vi "Open Class.vi"(6 "Variant in":variant, 7 "Shift Pressed?":bool, 8 "error in (no error)":errorcluster, 10 "QD Combo Box Ref":refnum<vi>, 11 "QD Launch VI Ref":refnum<vi>) -> (0 "error out":errorcluster, 4 "Variant out":variant)   [LabVIEW 2020]
doc: "Finds a class in the selection (wire, terminal, control, subVI, etc), and opens it. If nothing is selected it opens the current VI's library.\n\nDefault Shortcut - [O]"
uses:
  <vilib>/Utility/traverseref.llb/VI Scripting - Traverse.lvlib
  <vilib>/Utility/traverseref.llb/TRef TravTarget.ctl
panel:
  # "Do not change the connector pane of this VI.\n\nSee the block diagram for directions on how to use this template."
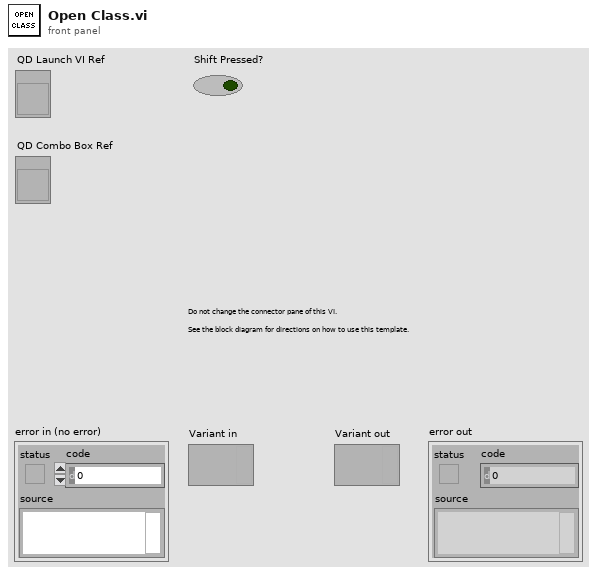
[diagram p1: front panel]
types:
  T1 = typedef "TRef TravTarget.ctl" = enum16{"FP", "BD", "Other"}
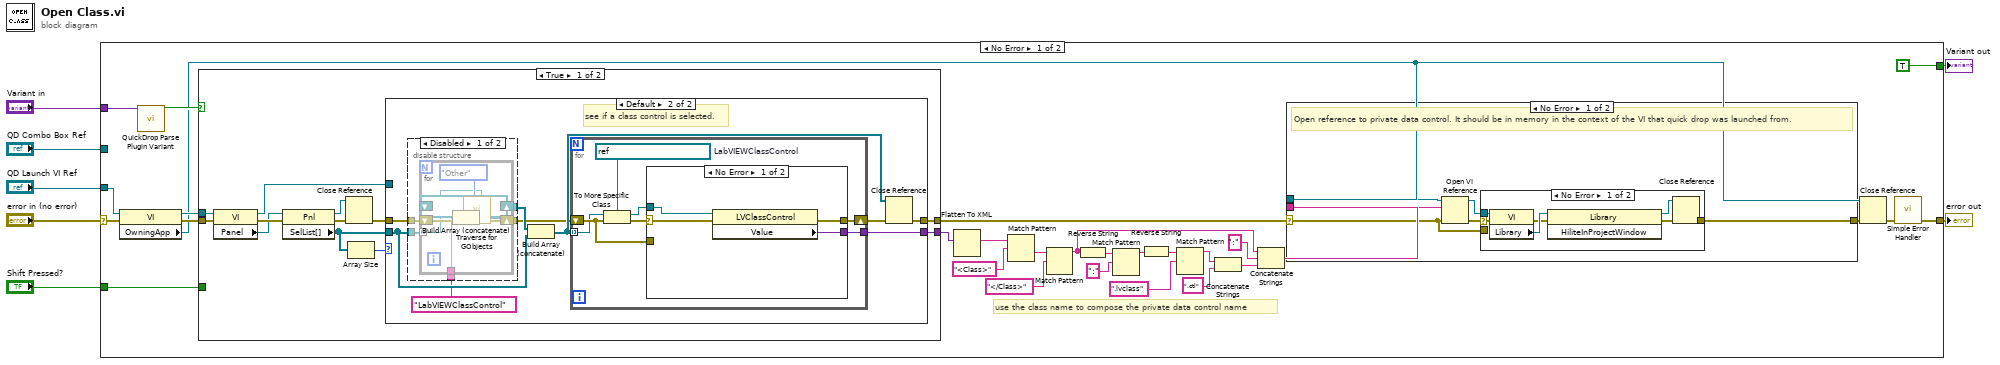
[diagram p0: block diagram]
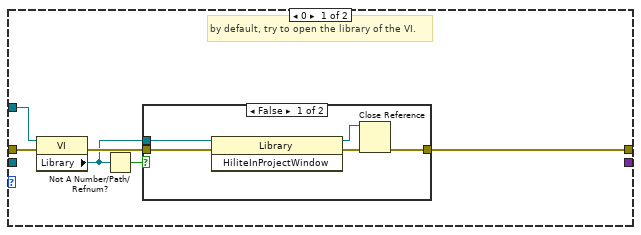
[diagram p4: hidden frame]
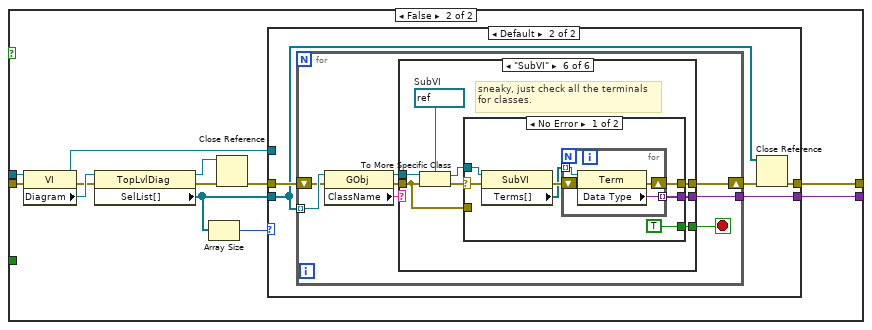
[diagram p8: hidden frame]
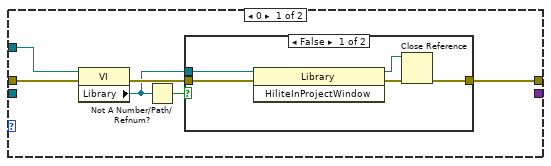
[diagram p9: hidden frame]
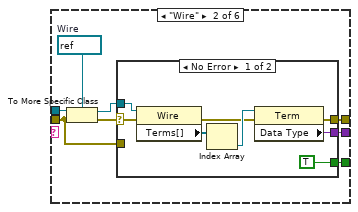
[diagram p12: hidden frame]
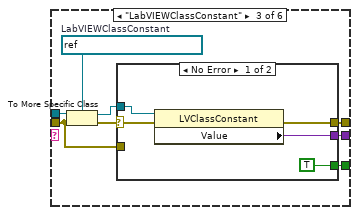
[diagram p14: hidden frame]
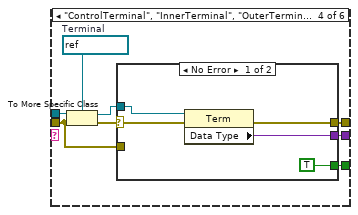
[diagram p16: hidden frame]
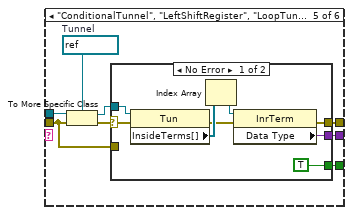
[diagram p18: hidden frame]
diagram:
  n1 = case shown="No Error" "error in (no error)" {
    selector: "error in (no error)" -> [w30 w232]
    tunnel: [w27 w232] -> w6
    tunnel: "QD Launch VI Ref" -> [w32 _]
    tunnel: "Shift Pressed?" -> [w34 _]
    tunnel: "QD Combo Box Ref" -> [_ _]
    tunnel: "Variant in" -> [w36 _]
    tunnel: [TRUE _] -> w1
    frame No Error {
      # "use the class name to compose the private data control name"
      n2 = property class="VI"(reference=w32, error in=w30) -> (reference out=w31:refnum<vi>, error out=w29:errorcluster, "OwningApp"=w8:refnum<vi>)
      n3 = call <vilib>:"QuickDrop Parse Plugin Variant.vi"("QDKS Variant in"=w36) -> ("QD Launch VI Panel?"=w33:bool)  [unwired: 12 in, 2 out]
      n4 = case shown="True" w33 {
        tunnel: w29 -> [w63 w123]
        tunnel: [w62 w122] -> w10
        tunnel: w34 -> [_ _]
        tunnel: w31 -> [w61 w121]
        tunnel: [w58 w116] -> w11
        frame True {
          n5 = property class="VI"(reference=w61, error in=w63) -> (reference out=w55:refnum<vi>, error out=w60:errorcluster, "Panel"=w59:refnum<vi>)
          n6 = property class="Pnl"(reference=w59, error in=w60) -> (reference out=w54:refnum<vi>, error out=w53:errorcluster, "SelList[]"=w56:refnum<vi>[])
          n7 = Close Reference(reference=w54, error in (no error)=w53) -> (error out=w52:errorcluster)
          n8 = Array Size(array=w56) -> (size(s)=w57:i32)
          n9 = case shown="Default" w57 {
            tunnel: [w65 w84] -> w62
            tunnel: w52 -> [w68 w82]
            tunnel: w56 -> [_ w80]
            tunnel: [_ w77] -> w58
            tunnel: w55 -> [w69 _]
            frame 0 {
              # "by default, try to open the library of the VI."
              n10 = property class="VI"(reference=w69, error in=w68) -> (error out=w66:errorcluster, "Library"=w64:refnum<vi>)  [unwired: 1 out]
              n11 = Not A Number/Path/Refnum?(number/path/refnum=w64) -> (NaN/Path/Refnum?=w67:bool)
              n12 = case shown="False" w67 {
                tunnel: w66 -> [w74 w75]
                tunnel: [w71 w75] -> w65
                tunnel: w64 -> [w70 _]
                frame False {
                  n13 = invoke class="Library" method="HiliteInProjectWindow"(reference=w70, error in=w74) -> (reference out=w72:refnum<vi>, error out=w73:errorcluster)  [unwired: 1 in, 1 out]
                  n14 = Close Reference(reference=w72, error in (no error)=w73) -> (error out=w71:errorcluster)
                }
                frame True {
                }
              }
            }
            frame Default {
              # "see if a class control is selected."
              n15 = disable-structure shown="Disabled" {
                disable-tunnel: [w90 w99] -> w76
                disable-tunnel: w82 -> [w89 w99]
                disable-tunnel: [w88 _] -> w81
                disable-tunnel: w80 -> [w87 _]
                disable-tunnel: "LabVIEWClassControl" ("Class Name") -> [w86 _]
                frame Disabled {
                  n16 = for {
                    shift-right: [w96] -> w90
                    shift-left: w89 -> [w95]
                    tunnel: w87 -> [w94] mode=indexing
                    tunnel: w86 -> [w93]
                    shift-right: [w91] -> w88
                    shift-left: refnum<vi>[] [] ("References") -> [w92]
                    n17 = call <vilib>:"Traverse for GObjects.vi"("Other Refnum"=w94, "Traverse Target"=TRef_TravTarget."Other", "error in (no error)"=w95, "Class Name"=w93) -> ("error out"=w96:errorcluster, "References"=w97:refnum<vi>[])  [unwired: 4 in, 2 out]
                    n18 = Build Array (concatenate)(w92, w97) -> (w91:refnum<vi>[])
                  }
                }
                frame Enabled {
                }
              }
              n19 = Build Array (concatenate)(w81, w80) -> (w83:refnum<vi>[])
              n20 = for {
                shift-right: [w106] -> w78
                shift-left: w76 -> [w103]
                tunnel: w83 -> [w102] mode=indexing
                tunnel: [w100] -> w77
                w101 = refnum<vi> refnum  # LabVIEWClassControl
                n21 = To More Specific Class(target class=w101, reference=w102, error in=w103) -> (specific class reference=w105:refnum<vi>, error out=w104:errorcluster)
                n22 = case shown="No Error" w104 {
                  selector: w104 -> [w110 _]
                  tunnel: [w109 w111] -> w106
                  tunnel: w105 -> [w108 _]
                  tunnel: w103 -> [_ w111]
                  tunnel: [w107 _] -> w100
                  frame No Error {
                    n23 = property class="LVClassControl"(reference=w108, error in=w110) -> (error out=w109:errorcluster, "Value"=w107:variant)  [unwired: 1 out]
                  }
                  frame Error {
                  }
                }
              }
              n24 = Close Reference(reference=w83, error in (no error)=w78) -> (error out=w84:errorcluster)
            }
          }
        }
        frame False {
          n25 = property class="VI"(reference=w121, error in=w123) -> (reference out=w112:refnum<vi>, error out=w119:errorcluster, "Diagram"=w120:refnum<vi>)
          n26 = property class="TopLvlDiag"(reference=w120, error in=w119) -> (reference out=w118:refnum<vi>, error out=w115:errorcluster, "SelList[]"=w114:refnum<vi>[])
          n27 = Array Size(array=w114) -> (size(s)=w113:i32)
          n28 = Close Reference(reference=w118, error in (no error)=w115) -> (error out=w117:errorcluster)
          n29 = case shown="Default" w113 {
            tunnel: [w126 w140] -> w122
            tunnel: w117 -> [w127 w139]
            tunnel: [_ w137] -> w116
            tunnel: w114 -> [_ w136]
            tunnel: w112 -> [w125 _]
            frame 0 {
              n30 = property class="VI"(reference=w125, error in=w127) -> (error out=w129:errorcluster, "Library"=w128:refnum<vi>)  [unwired: 1 out]
              n31 = Not A Number/Path/Refnum?(number/path/refnum=w128) -> (NaN/Path/Refnum?=w124:bool)
              n32 = case shown="False" w124 {
                tunnel: w129 -> [w134 w135]
                tunnel: [w131 w135] -> w126
                tunnel: w128 -> [w130 _]
                frame False {
                  n33 = invoke class="Library" method="HiliteInProjectWindow"(reference=w130, error in=w134) -> (reference out=w132:refnum<vi>, error out=w133:errorcluster)  [unwired: 1 in, 1 out]
                  n34 = Close Reference(reference=w132, error in (no error)=w133) -> (error out=w131:errorcluster)
                }
                frame True {
                }
              }
            }
            frame Default {
              n35 = for {
                shift-right: [w148] -> w138
                shift-left: w139 -> [w144]
                tunnel: w136 -> [w145] mode=indexing
                tunnel: [w146] -> w137
                stop <- w147 stop-if-true
                n36 = property class="GObj"(reference=w145, error in=w144) -> (reference out=w142:refnum<vi>, error out=w143:errorcluster, "ClassName"=w141:string)
                n37 = case shown="\"SubVI\"" w141 {
                  tunnel: [w149 w155 w173 w187 w201 w218] -> w148
                  tunnel: [_ w153 w171 w185 w199 w216] -> w147
                  tunnel: [_ w152 w170 w184 w198 w215] -> w146
                  tunnel: w143 -> [w149 w151 w169 w183 w197 w214]
                  tunnel: w142 -> [_ w150 w168 w182 w196 w213]
                  frame Default {
                  }
                  frame "Wire" {
                    w157 = refnum<vi> refnum  # Wire
                    n38 = To More Specific Class(target class=w157, reference=w150, error in=w151) -> (specific class reference=w154:refnum<vi>, error out=w156:errorcluster)
                    n39 = case shown="No Error" w156 {
                      selector: w156 -> [w165 _]
                      tunnel: [w160 w166] -> w155
                      tunnel: w154 -> [w164 _]
                      tunnel: w151 -> [_ w166]
                      tunnel: [TRUE _] -> w153
                      tunnel: [w158 _] -> w152
                      frame No Error {
                        n40 = property class="Wire"(reference=w164, error in=w165) -> (error out=w161:errorcluster, "Terms[]"=w163:refnum<vi>[])  [unwired: 1 out]
                        n41 = Index Array(array=w163) -> (element=w162:refnum<vi>)  [unwired: 1 in]
                        n42 = property class="Term"(reference=w162, error in=w161) -> (error out=w160:errorcluster, "Data Type"=w158:variant)  [unwired: 1 out]
                      }
                      frame Error {
                      }
                    }
                  }
                  frame "LabVIEWClassConstant" {
                    w167 = refnum<vi> refnum  # LabVIEWClassConstant
                    n43 = To More Specific Class(target class=w167, reference=w168, error in=w169) -> (specific class reference=w172:refnum<vi>, error out=w174:errorcluster)
                    n44 = case shown="No Error" w174 {
                      selector: w174 -> [w177 _]
                      tunnel: [w176 w180] -> w173
                      tunnel: w172 -> [w178 _]
                      tunnel: w169 -> [_ w180]
                      tunnel: [TRUE _] -> w171
                      tunnel: [w175 _] -> w170
                      frame No Error {
                        n45 = property class="LVClassConstant"(reference=w178, error in=w177) -> (error out=w176:errorcluster, "Value"=w175:variant)  [unwired: 1 out]
                      }
                      frame Error {
                      }
                    }
                  }
                  frame "ControlTerminal", "InnerTerminal", "OuterTerminal", "Terminal" {
                    w181 = refnum<vi> refnum  # Terminal
                    n46 = To More Specific Class(target class=w181, reference=w182, error in=w183) -> (specific class reference=w186:refnum<vi>, error out=w188:errorcluster)
                    n47 = case shown="No Error" w188 {
                      selector: w188 -> [w191 _]
                      tunnel: [w190 w194] -> w187
                      tunnel: w186 -> [w192 _]
                      tunnel: w183 -> [_ w194]
                      tunnel: [TRUE _] -> w185
                      tunnel: [w189 _] -> w184
                      frame No Error {
                        n48 = property class="Term"(reference=w192, error in=w191) -> (error out=w190:errorcluster, "Data Type"=w189:variant)  [unwired: 1 out]
                      }
                      frame Error {
                      }
                    }
                  }
                  frame "ConditionalTunnel", "LeftShiftRegister", "LoopTunnel", "RegionTunnel", "RightShiftRegister", "SelectorTunnel", "Tunnel" {
                    w195 = refnum<vi> refnum  # Tunnel
                    n49 = To More Specific Class(target class=w195, reference=w196, error in=w197) -> (specific class reference=w200:refnum<vi>, error out=w202:errorcluster)
                    n50 = case shown="No Error" w202 {
                      selector: w202 -> [w208 _]
                      tunnel: [w203 w211] -> w201
                      tunnel: w200 -> [w209 _]
                      tunnel: w197 -> [_ w211]
                      tunnel: [TRUE _] -> w199
                      tunnel: [w205 _] -> w198
                      frame No Error {
                        n51 = property class="Tun"(reference=w209, error in=w208) -> (error out=w204:errorcluster, "InsideTerms[]"=w207:refnum<vi>[])  [unwired: 1 out]
                        n52 = Index Array(array=w207) -> (element=w206:refnum<vi>)  [unwired: 1 in]
                        n53 = property class="InrTerm"(reference=w206, error in=w204) -> (error out=w203:errorcluster, "Data Type"=w205:variant)  [unwired: 1 out]
                      }
                      frame Error {
                      }
                    }
                  }
                  frame "SubVI" {
                    w212 = refnum<vi> refnum  # SubVI
                    # "sneaky, just check all the terminals\nfor classes."
                    n54 = To More Specific Class(target class=w212, reference=w213, error in=w214) -> (specific class reference=w217:refnum<vi>, error out=w219:errorcluster)
                    n55 = case shown="No Error" w219 {
                      selector: w219 -> [w224 _]
                      tunnel: [w221 w231] -> w218
                      tunnel: w217 -> [w225 _]
                      tunnel: w214 -> [_ w231]
                      tunnel: [TRUE _] -> w216
                      tunnel: [w223 _] -> w215
                      frame No Error {
                        n56 = property class="SubVI"(reference=w225, error in=w224) -> (error out=w222:errorcluster, "Terms[]"=w220:refnum<vi>[])  [unwired: 1 out]
                        n57 = for {
                          tunnel: [w230] -> w223 mode=indexing
                          shift-right: [w228] -> w221
                          shift-left: w222 -> [w229]
                          tunnel: w220 -> [w227] mode=indexing
                          n58 = property class="Term"(reference=w227, error in=w229) -> (error out=w228:errorcluster, "Data Type"=w230:variant)  [unwired: 1 out]
                        }
                      }
                      frame Error {
                      }
                    }
                  }
                }
              }
              n59 = Close Reference(reference=w136, error in (no error)=w138) -> (error out=w140:errorcluster)
            }
          }
        }
      }
      n60 = Flatten To XML(6:w11) -> (2:w19:string)
      n61 = Match Pattern(string=w19, regular expression="<Class>") -> (after substring=w24:string)  [unwired: 1 in, 3 out]
      n62 = Match Pattern(string=w24, regular expression="</Class>") -> (before substring=w18:string)  [unwired: 1 in, 3 out]
      n63 = Reverse String(1:w18) -> (0:w22:string)
      n64 = Match Pattern(string=w22, regular expression=":") -> (before substring=w20:string)  [unwired: 1 in, 3 out]
      n65 = Reverse String(1:w20) -> (0:w16:string)
      n66 = Match Pattern(string=w16, regular expression=".lvclass") -> (before substring=w13:string)  [unwired: 1 in, 3 out]
      n67 = Concatenate Strings(w13, ".ctl" ("string")) -> (w12:string)
      n68 = Concatenate Strings(w18, ":" ("regular expression"), w12) -> (w26:string)
      n69 = case shown="No Error" w10 {
        selector: w10 -> [w37 w51]
        tunnel: w26 -> [w42 _]
        tunnel: [w39 w51] -> w9
        tunnel: w8 -> [w38 _]
        frame No Error {
          # "Open reference to private data control. It should be in memory in the context of the VI that quick drop was launched from."
          n70 = Open VI Reference(application reference (local)=w38, vi path=w42, error in (no error)=w37) -> (vi reference=w41:refnum<vi>, error out=w40:errorcluster)  [unwired: 3 in]
          n71 = case shown="No Error" w40 {
            selector: w40 -> [w48 _]
            tunnel: w41 -> [w49 _]
            tunnel: [w43 w50] -> w39
            tunnel: w37 -> [_ w50]
            frame No Error {
              n72 = property class="VI"(reference=w49, error in=w48) -> (error out=w46:errorcluster, "Library"=w47:refnum<vi>)  [unwired: 1 out]
              n73 = invoke class="Library" method="HiliteInProjectWindow"(reference=w47, error in=w46) -> (reference out=w44:refnum<vi>, error out=w45:errorcluster)  [unwired: 1 in, 1 out]
              n74 = Close Reference(reference=w44, error in (no error)=w45) -> (error out=w43:errorcluster)
            }
            frame Error {
            }
          }
        }
        frame Error {
        }
      }
      n75 = Close Reference(reference=w8, error in (no error)=w9) -> (error out=w28:errorcluster)
      n76 = call <vilib>:"Simple Error Handler.vi"("error in (no error)"=w28) -> ("error out"=w27:errorcluster)  [unwired: 4 in, 4 out]
    }
    frame Error {
    }
  }
  "error out" <- w6
  "Variant out" <- w1
